vi "Configure Measurement Type.vi"(0 "VISA resource name":refnum<visa-resource-name>, 1 "Enable Clear (F: Disable)":bool, 2 "Enable Statistics Reset (F: Disable)":bool, 5 "Measurement Type (0: Peak-Peak)":i32(ring) items=["Peak-Peak", "Maximum", "Minimum", "Amplitude", "Top", "Base", "Overshoot", "Preshoot", "Average - N Cycles", "Average - Full Screen", "DC RMS - N Cycles", "DC RMS - Full Screen", "AC RMS - N Cycles", "AC RMS - Full Screen (Std Dev)", "Ratio", "Period", "Frequency", "Counter", "+Width", "-Width", "Burst Width", "Duty Cycle", "Rise Time", "Fall Time", "Delay", "Phase", "X minY", "X maxY", "Positive Pulse Count", "Negative Pulse Count", "Raising Edge Count", "Falling Edge Count", "Area - N Cycle", "Area - Full Screen", "Bit Rate", "Negative Duty Cycle", "Standard Deviation"], 7 "Measurement Source 1 (0: Channel 1)":i32(ring) items=["Channel 1"=0, "Channel 2"=1, "Channel 3"=2, "Channel 4"=3, "Waveform Memory 1"=5, "Waveform Memory 2"=6, "Serial Bus 1"=7, "Serial Bus 2"=8, "Digital Bus Low"=9, "Digital Bus High "=10, "Digital Bus 1"=11, "Digital Bus 2"=12, "D0"=13, "D1"=14, "D2"=15, "D3"=16, "D4"=17, "D5"=18, "D6"=19, "D7"=20, "D8"=21, "D9"=22, "D10"=23, "D11"=24, "D12"=25, "D13"=26, "D14"=27, "D15"=28, "External"=29, "Function 1"=32, "Function 2"=33, "Function 3"=34, "Function 4"=35, "Math 1"=36, "Math 2"=37, "Math 3"=38, "Math 4"=39, "FFT"=40, "Analog Bus"=41], 9 "Measurement Source 2 (1: Channel 2)":i32(ring)=1 items=["Channel 1", "Channel 2", "Channel 3", "Channel 4", "Math1", "Math2", "Math3", "Math4", "Waveform Memory 1", "Waveform Memory 2", "Function 1", "Function 2", "Function 3", "Function 4"], 11 "error in (no error)":errorcluster) -> (4 "VISA resource name out":refnum<visa-resource-name>, 15 "error out":errorcluster)   [LabVIEW 2017, in "Agilent 2000 3000 X-Series.lvlib"]
doc: "Configures the measurement type."
uses:
  Agilent 2000 3000 X-Series.lvlib
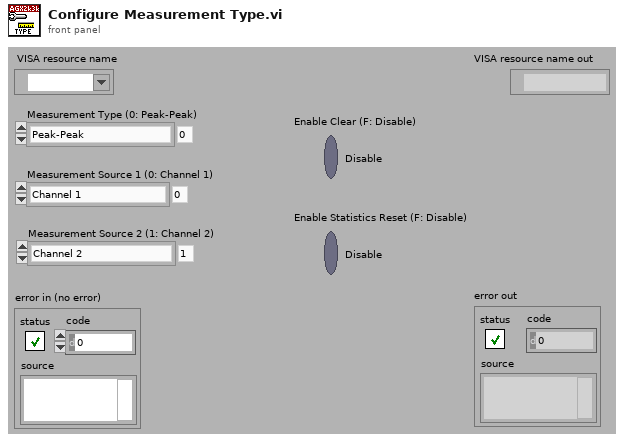
[diagram p1: front panel]
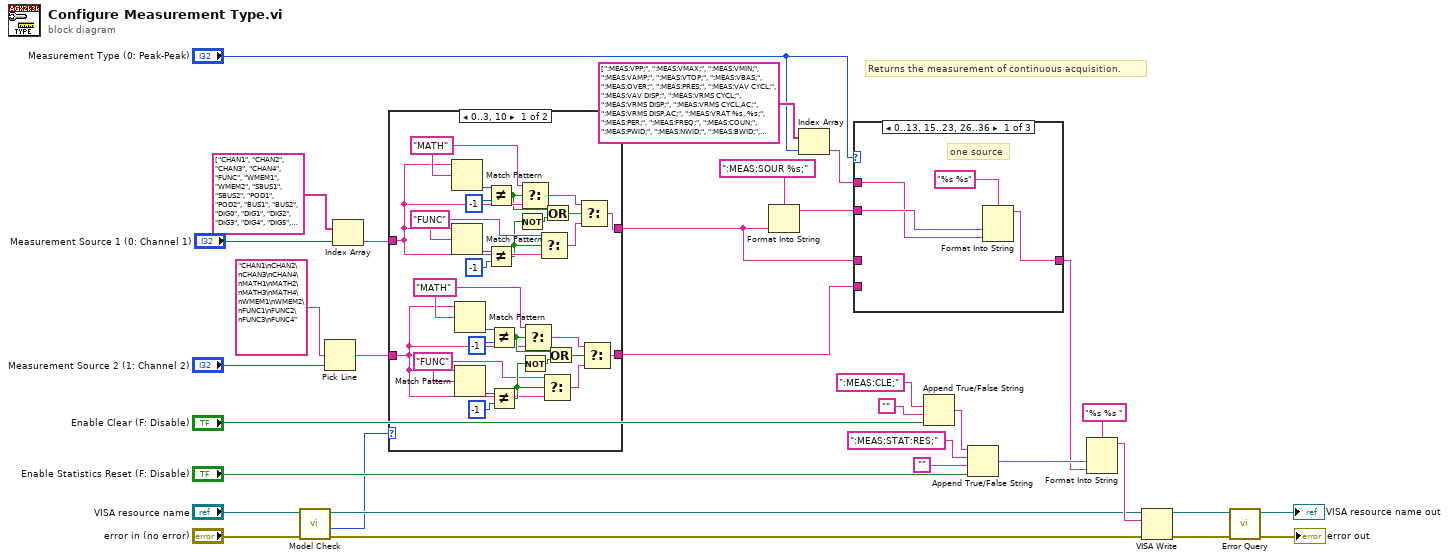
[diagram p0: block diagram]
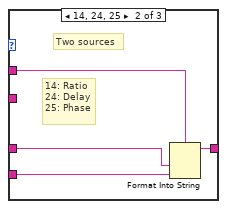
[diagram p3: hidden frame]
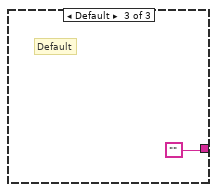
[diagram p4: hidden frame]
diagram:
  # "Returns the measurement of continuous acquisition."
  n1 = call "Model Check.vi"("error in (no error)"="error in (no error)", "VISA resource name"="VISA resource name") -> ("error out"=w4:errorcluster, "Model"=w3:i32, "VISA resource name out"=w5:refnum<visa-resource-name>)  [unwired: 6 in, 1 out]
  n2 = Pick Line(multi-line string="CHAN1\nCHAN2\nCHAN3\nCHAN4\nMATH1\nMATH2\nMATH3\nMATH4\nWMEM1\nWMEM2\nFUNC1\nFUNC2\nFUNC3\nFUNC4", line index="Measurement Source 2 (1: Channel 2)") -> (output string=w2:string)  [unwired: 1 out]
  n3 = Index Array(array=string[] ["CHAN1", "CHAN2", "CHAN3", "CHAN4", "FUNC", "WMEM1", "WMEM2", "SBUS1", "SBUS2", "POD1", "POD2", "BUS1", "BUS2", "DIG0", "DIG1", "DIG2", "DIG3", "DIG4", "DIG5", "DIG6", "DIG7", "DIG8", "DIG9", "DIG10", "DIG11", "DIG12", "DIG13", "DIG14", "DIG15", "EXT", "LINE", "WGEN", "FUNC1", "FUNC2", "FUNC3", "FUNC4", "MATH1", "MATH2", "MATH3", "MATH4", "FFT", "ABUS"], index="Measurement Source 1 (0: Channel 1)") -> (element=w9:string)
  n4 = case shown="0..3, 10" w3 {
    tunnel: w9 -> [w56 w63]
    tunnel: [w52 w63] -> w8
    tunnel: w2 -> [w35 w62]
    tunnel: [w34 w62] -> w1
    frame 0..3, 10 {
      w41 = "FUNC" ("regular expression")
      w38 = "MATH" ("regular expression")
      w55 = "FUNC" ("regular expression")
      w59 = "MATH" ("regular expression")
      n5 = Match Pattern(string=w56, regular expression=w59) -> (offset past match=w61:i32)  [unwired: 1 in, 3 out]
      n6 = Match Pattern(string=w56, regular expression=w55) -> (offset past match=w58:i32)  [unwired: 1 in, 3 out]
      n7 = Match Pattern(string=w35, regular expression=w38) -> (offset past match=w36:i32)  [unwired: 1 in, 3 out]
      n8 = Match Pattern(string=w35, regular expression=w41) -> (offset past match=w39:i32)  [unwired: 1 in, 3 out]
      n9 = Not Equal?(x=w61, y=-1) -> (x != y?=w50:bool)
      n10 = Not Equal?(x=w58, y=-1) -> (x != y?=w48:bool)
      n11 = Not Equal?(x=w36, y=-1) -> (x != y?=w45:bool)
      n12 = Not Equal?(x=w39, y=-1) -> (x != y?=w47:bool)
      n13 = Not(x=w48) -> (.not. x?=w49:bool)
      n14 = Select(t=w59, s=w50, f=w56) -> (s? t:f=w54:string)
      n15 = Not(x=w47) -> (.not. x?=w46:bool)
      n16 = Select(t=w38, s=w45, f=w35) -> (s? t:f=w42:string)
      n17 = Select(t=w55, s=w48, f=w56) -> (s? t:f=w53:string)
      n18 = Select(t=w41, s=w47, f=w35) -> (s? t:f=w43:string)
      n19 = Or(x=w50, y=w49) -> (x .or. y?=w51:bool)
      n20 = Or(x=w45, y=w46) -> (x .or. y?=w44:bool)
      n21 = Select(t=w54, s=w51, f=w53) -> (s? t:f=w52:string)
      n22 = Select(t=w42, s=w44, f=w43) -> (s? t:f=w34:string)
    }
    frame Default {
    }
  }
  n23 = Format Into String(format string=":MEAS:SOUR %s;", w8) -> (resulting string=w30:string)  [unwired: 2 in, 1 out]
  n24 = Index Array(array=string[] [":MEAS:VPP;", ":MEAS:VMAX;", ":MEAS:VMIN;", ":MEAS:VAMP;", ":MEAS:VTOP;", ":MEAS:VBAS;", ":MEAS:OVER;", ":MEAS:PRES;", ":MEAS:VAV CYCL;", ":MEAS:VAV DISP;", ":MEAS:VRMS CYCL;", ":MEAS:VRMS DISP;", ":MEAS:VRMS CYCL,AC;", ":MEAS:VRMS DISP,AC;", ":MEAS:VRAT %s, %s;", ":MEAS:PER;", ":MEAS:FREQ;", ":MEAS:COUN;", ":MEAS:PWID;", ":MEAS:NWID;", ":MEAS:BWID;", ":MEAS:DUTY;", ":MEAS:RIS;", ":MEAS:FALL;", ":MEAS:DEL %s, %s;", ":MEAS:PHAS %s, %s;", ":MEAS:XMIN;", ":MEAS:XMAX;", ":MEAS:PPUL;", ":MEAS:NPUL;", ":MEAS:PEDG;", ":MEAS:NEDG;", ":MEAS:ARE CYCL;", ":MEAS:ARE DISP;", ":MEAS:BRAT", ":MEAS:NDUT", ":MEAS:SDEV", "", ""] ("Array"), index="Measurement Type (0: Peak-Peak)") -> (element=w14:string)
  n25 = case shown="0..13, 15..23, 26..36" "Measurement Type (0: Peak-Peak)" {
    tunnel: w8 -> [_ w71 _]
    tunnel: w1 -> [_ w70 _]
    tunnel: [w64 w69 ""] -> w23
    tunnel: w30 -> [w66 _ _]
    tunnel: w14 -> [w65 w68 _]
    frame 0..13, 15..23, 26..36 {
      # "one source"
      n26 = Format Into String(format string="%s %s", w66, w65) -> (resulting string=w64:string)  [unwired: 2 in, 1 out]
    }
    frame 14, 24, 25 {
      # "14: Ratio\n24: Delay\n25: Phase"
      # "Two sources"
      n27 = Format Into String(format string=w68, w71, w70) -> (resulting string=w69:string)  [unwired: 2 in, 1 out]
    }
    frame Default {
      # "Default"
    }
  }
  n28 = Append True/False String(1:"Enable Clear (F: Disable)", 2:"", 3:":MEAS:CLE;") -> (0:w22:string)  [unwired: 1 out]
  n29 = Append True/False String(1:"Enable Statistics Reset (F: Disable)", 2:"", 3:":MEAS:STAT:RES;", 4:w22) -> (0:w24:string)
  n30 = Format Into String(format string="%s %s ", w24, w23) -> (resulting string=w15:string)  [unwired: 2 in, 1 out]
  n31 = VISA Write(VISA resource name=w5, write buffer=w15, error in (no error)=w4) -> (VISA resource name out=w19:refnum<visa-resource-name>, error out=w18:errorcluster)  [unwired: 1 out]
  n32 = call "Error Query.vi"("error in (no error)"=w18, "VISA resource name"=w19) -> ("error out"=→"error out":errorcluster, "VISA resource name out"=→"VISA resource name out":refnum<visa-resource-name>)  [unwired: 8 out]
